vi "PositionerCapture.vi"() -> ()   [LabVIEW 2011]
doc: "CONEX - CC Virtual Front Panel:\n\nThis is a sample of an application that can be built with the LabVIEW drivers.\n\nPress HOME / ENABLE in top left of panel to put stage in Ready state for motion."
uses:
  <vilib>/userDefined/High Color/IMAQdx.ctl
  <vilib>/Platform/TimedLoop/XDataNode/timing_clust.ctl
  <vilib>/Platform/TimedLoop/XDataNode/nitl_modes.ctl
  <vilib>/Platform/TimedLoop/XDataNode/wakeup.ctl
  <vilib>/Platform/TimedLoop/XDataNode/XDataNode.xnode
  <vilib>/Platform/TimedLoop/XDataNode/XDNodeRunTimeDep.lvlib
  <vilib>/vision/driver/NI_Vision_Acquisition_Software.lvlib
panel:
  out "Current noUnits":dbl caption="mm" format="%#_6f"
  in  "lambda":dbl caption="nm" format="%#_6f"
  in  "Units":string(combo)="mm"
  in  "Go0":bool
  in  "Zero position":dbl caption="um" format="%#_6f"
  in  "Tare":bool
  out "Relative position":dbl caption="um" format="%#_6f"
  in  "Path to save the captures":path
  out "Image":T1(plugin-control)
  in  "(1) Go to:":dbl=1.0 caption="um"
  out "Title":string
  in  "Set Max":bool
  in  "Set Min":bool
  in  "Max":dbl
  in  "Min":dbl
  in  "Set velocity":bool
  out "Stop cycle":bool=TRUE
  out "Title 2":string
  in  "Cycle":bool
  in  "Go2":bool
  in  "Go1":bool
  in  "(2) Go to:":dbl=1.0 caption="um"
  in  "-":bool
  in  "+":bool
  in  "Step:":dbl caption="um" format="%#_6f"
  out "Position History":dbl(graph)=1.5
  in  "Action":bool
  out "Stop polling":bool=TRUE
  out "Controller state description":string="STATUS"
  out "Velocity MAX":dbl=0.4
  out "Controller state":string="33"
  out "Positioner error":string="0000"
  in  "Velocity:":dbl format="%#_6f"
  in  "Exit":bool=TRUE
  out "Target position":dbl
  in  "Exit":bool
  in  "Position glissière":cluster{dbl, dbl}(slide) scale=4.5..6.0
  out "Current position":dbl caption="um" format="%#_6f"
  # "mm/s"
  # "mm"
  # "Limits:"
  # "mm"
  # "(1)"
  # "(2)"
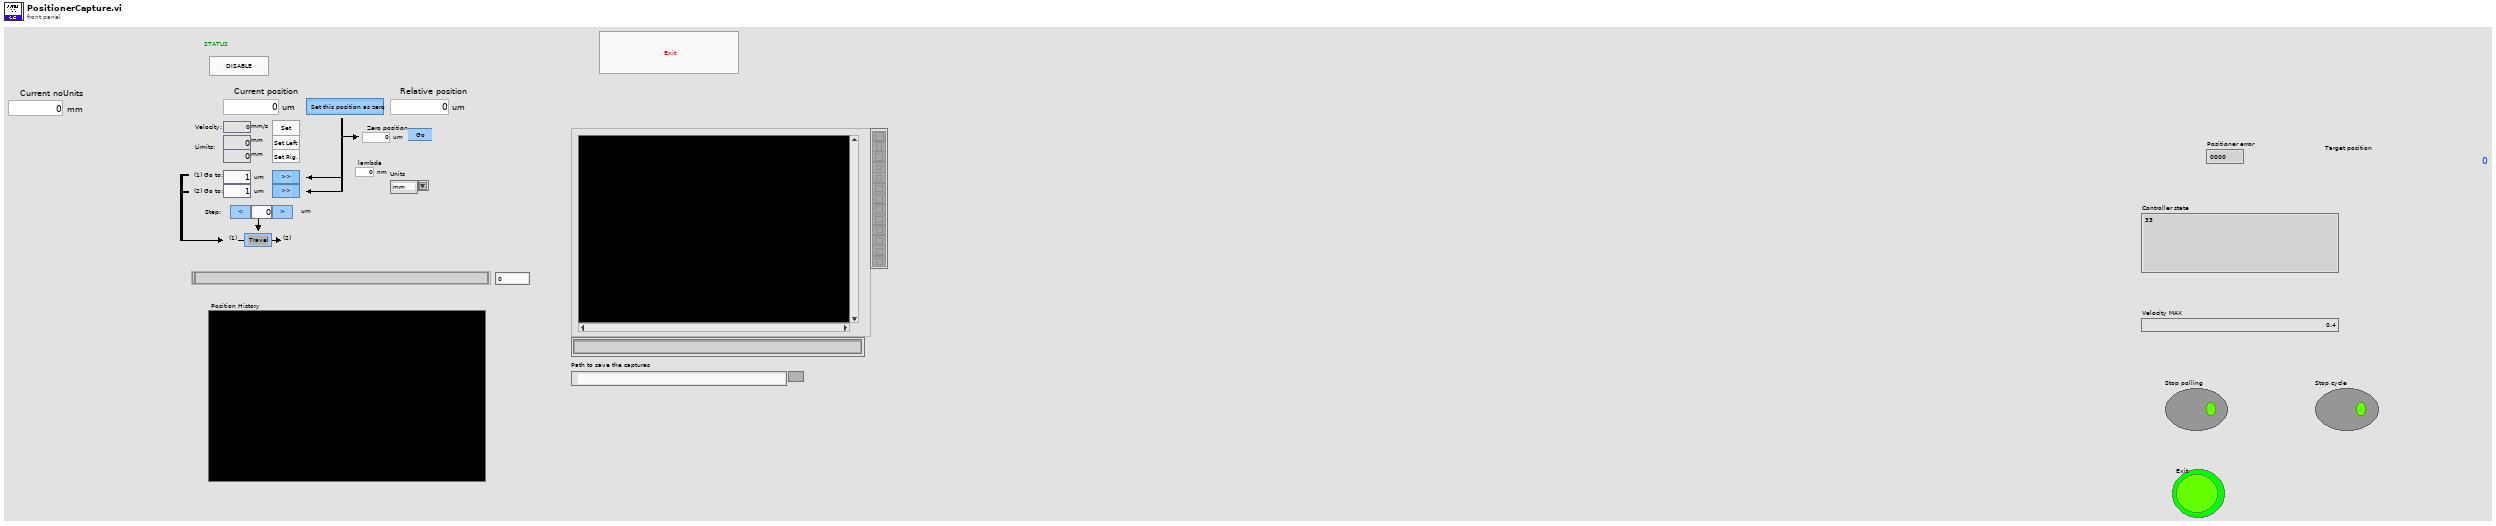
[diagram p1: front panel]
types:
  T1 = typedef "IMAQ Image.ctl" = refnum<image>
  T2 = typedef "IMAQdx.ctl" = refnum<k21>
  T3 = typedef "XDNodeRunTimeDep.lvlib/timing_clust.ctl" = cluster{"Expected End [f-1]":u64, "Actual End [f-1]":u64, "Finished Late? [f-1]":bool, "Expected End [i-1]":u64, "Actual End [i-1]":u64, "Finished Late? [i-1]":bool, "Expected Start [i]":u64, "Actual Start [i]":u64, "Expected Start [f]":u64, "Actual Start [f]":u64, "Source Name":string, "Structure Name":string, "Period":i64, "Deadline":i64, "Offset":i64, "Start":i64, "Priority":i32, "Timeout":i32, "Mode":T4, "Wakeup Reason":T5, "Error":errorcluster, "Source Type":string, "Secondary Source Type":string, "Global End Time":u64, "Global Start Time":u64, "Frame Duration":u64, "Iteration Duration":u64, "Assigned CPU":i32, "I/O Scan Engine Mode":u32}
  T4 = typedef "XDNodeRunTimeDep.lvlib/nitl_modes.ctl" = enum32{"No Change", "Process missed periods, maintain original phase", "Discard missed periods, maintain original phase", "Process missed periods, ignore original phase", "Discard missed periods, ignore original phase"}
  T5 = typedef "XDNodeRunTimeDep.lvlib/wakeup.ctl" = enum32{"Normal", "Aborted", "Asynchronous wakeup", "Timing source error", "Timed loop error", "Timeout"}
  T6 = cluster{"VISA resource name":refnum<visa-resource-name>, "Device name":string, "Controller address":i32, "error":errorcluster}
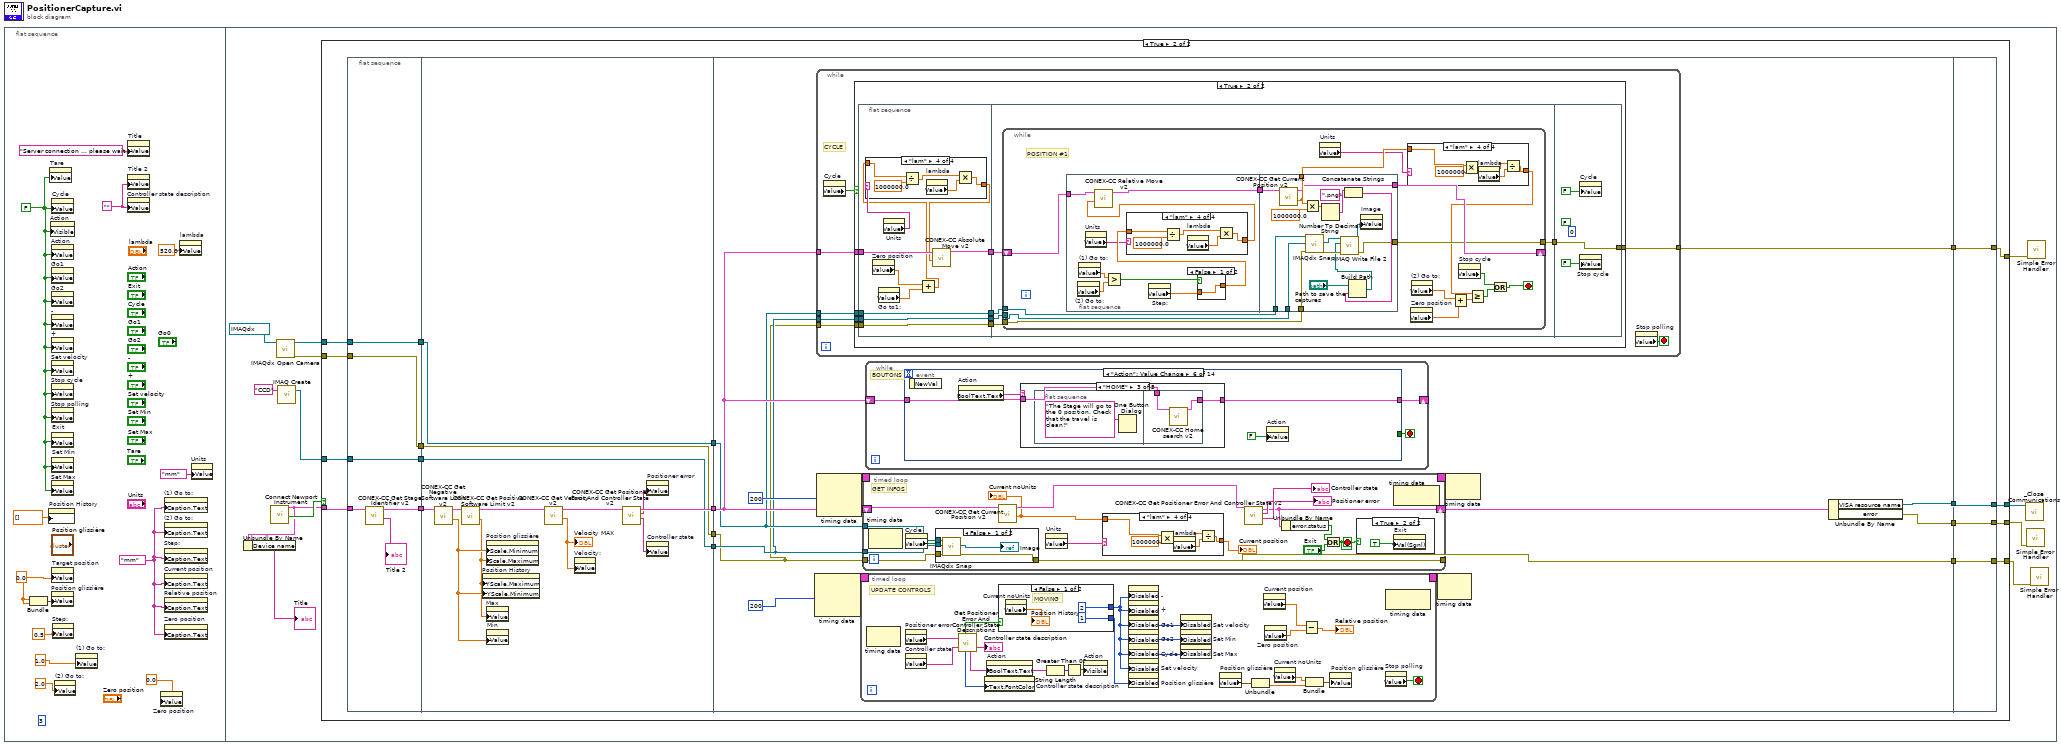
[diagram p0: block diagram]
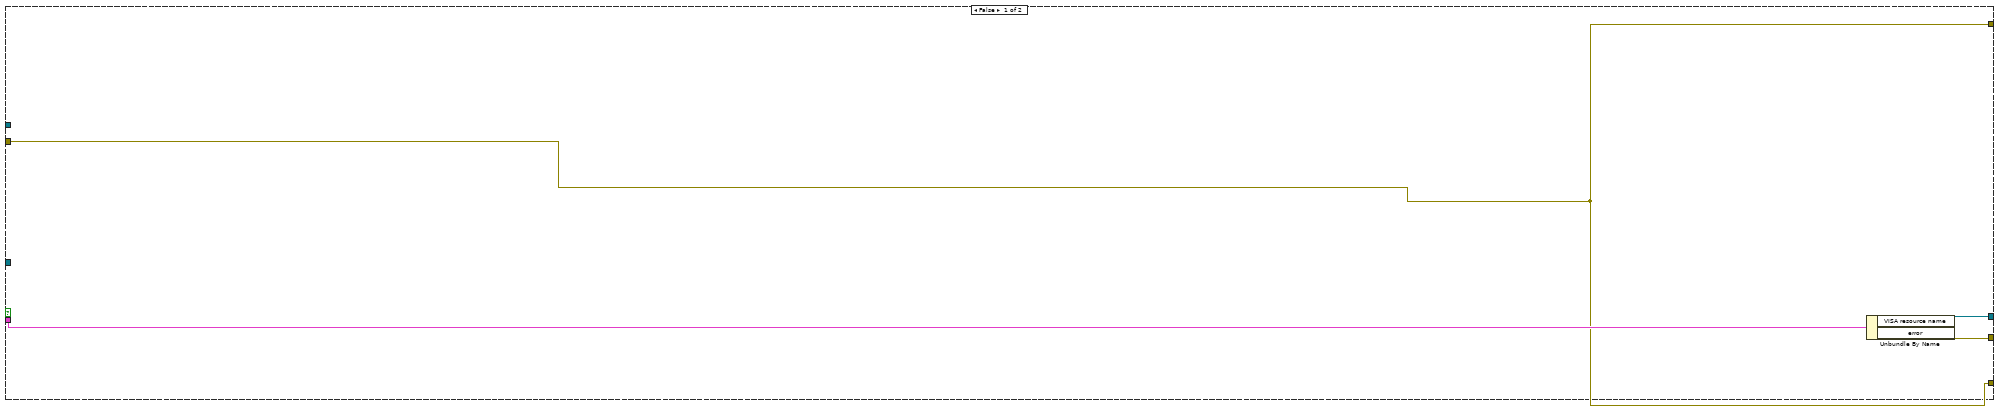
[diagram p2: hidden frame]
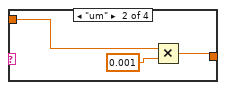
[diagram p5: hidden frame]
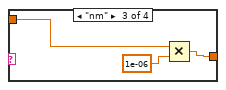
[diagram p6: hidden frame]
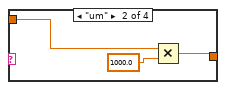
[diagram p8: hidden frame]
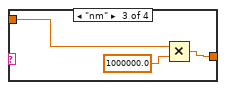
[diagram p9: hidden frame]
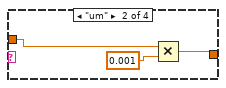
[diagram p11: hidden frame]
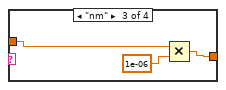
[diagram p12: hidden frame]
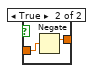
[diagram p13: hidden frame]
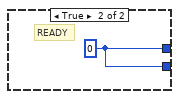
[diagram p14: hidden frame]
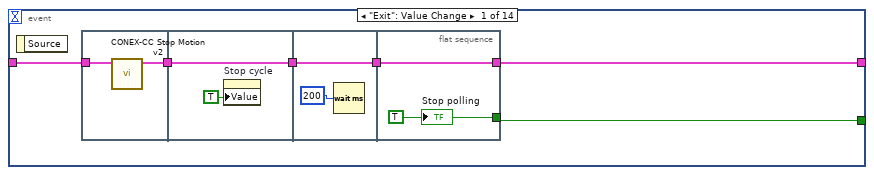
[diagram p15: hidden frame]
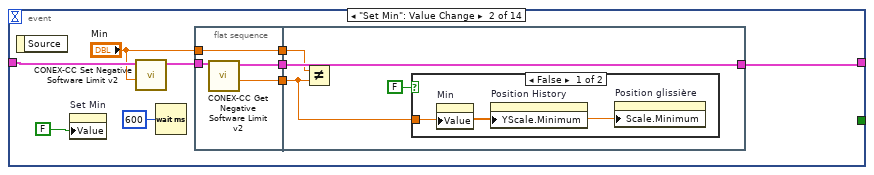
[diagram p16: hidden frame]
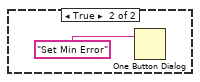
[diagram p17: hidden frame]
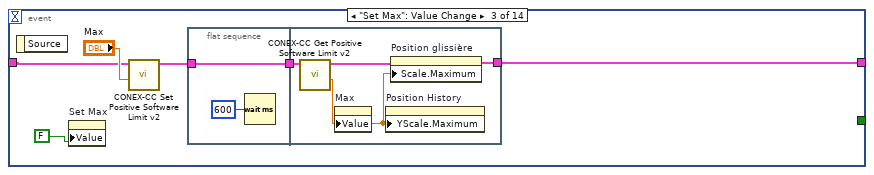
[diagram p18: hidden frame]
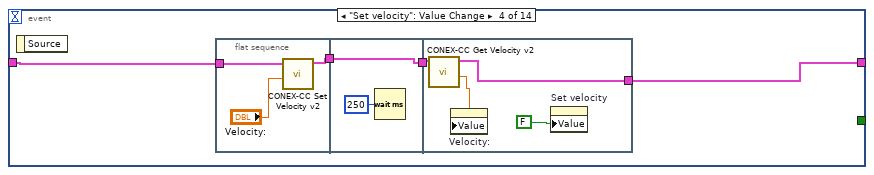
[diagram p19: hidden frame]
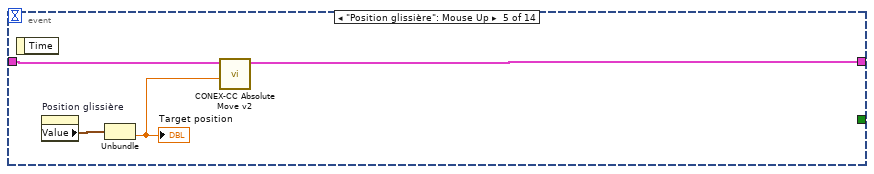
[diagram p20: hidden frame]
diagram:
  n1 = flat-sequence {
    frame #0 {
      w2 = "mm" ("Units")
      (unwired) 3 ("# Loops")
      w6 = FALSE
      w12 = 0.0
      w11 = ""
      n2 = Bundle(w12, w12) -> (w13:cluster{dbl, dbl})  [unwired: 1 out]
      n3 = property on="Position History" class="WFChart (strict)"("History Data"=dbl[] [] ("Données d'historique")) -> ()  [unwired: 2 in, 2 out]
      n4 = property on="Tare" class="Bool (strict)"("Value"=w6) -> ()  [unwired: 2 in, 2 out]
      n5 = property on="Action" class="Bool (strict)"("Visible"=w6) -> ()  [unwired: 2 in, 2 out]
      n6 = property on="Cycle" class="Bool (strict)"("Value"=w6) -> ()  [unwired: 2 in, 2 out]
      n7 = property on="Action" class="Bool (strict)"("Value"=w6) -> ()  [unwired: 2 in, 2 out]
      n8 = property on="Go1" class="Bool (strict)"("Value"=w6) -> ()  [unwired: 2 in, 2 out]
      n9 = property on="Go2" class="Bool (strict)"("Value"=w6) -> ()  [unwired: 2 in, 2 out]
      n10 = property on="-" class="Bool (strict)"("Value"=w6) -> ()  [unwired: 2 in, 2 out]
      n11 = property on="+" class="Bool (strict)"("Value"=w6) -> ()  [unwired: 2 in, 2 out]
      n12 = property on="Set velocity" class="Bool (strict)"("Value"=w6) -> ()  [unwired: 2 in, 2 out]
      n13 = property on="Stop cycle" class="Bool (strict)"("Value"=w6) -> ()  [unwired: 2 in, 2 out]
      n14 = property on="Stop polling" class="Bool (strict)"("Value"=w6) -> ()  [unwired: 2 in, 2 out]
      n15 = property on="Exit" class="Bool (strict)"("Value"=w6) -> ()  [unwired: 2 in, 2 out]
      n16 = property on="Set Min" class="Bool (strict)"("Value"=w6) -> ()  [unwired: 2 in, 2 out]
      n17 = property on="Set Max" class="Bool (strict)"("Value"=w6) -> ()  [unwired: 2 in, 2 out]
      n18 = property on="Target position" class="DigNum (strict)"("Value"=w12) -> ()  [unwired: 2 in, 2 out]
      n19 = property on="Position glissière" class="Slide (strict)"("Value"=w13) -> ()  [unwired: 2 in, 2 out]
      n20 = property on="Step:" class="DigNum (strict)"("Value"=0.5 ("Step")) -> ()  [unwired: 2 in, 2 out]
      n21 = property on="(2) Go to:" class="DigNum (strict)"("Value"=2.0 ("Abs. Move 2")) -> ()  [unwired: 2 in, 2 out]
      n22 = property on="(1) Go to:" class="DigNum (strict)"("Value"=1.0 ("Abs. Move 1")) -> ()  [unwired: 2 in, 2 out]
      n23 = property on="Title" class="Str"("Value"="Server connection ... please wait." ("Title")) -> ()  [unwired: 2 in, 2 out]
      n24 = property on="Title 2" class="Str"("Value"=w11) -> ()  [unwired: 2 in, 2 out]
      n25 = property on="Controller state description" class="Str"("Value"=w11) -> ()  [unwired: 2 in, 2 out]
      n26 = property on="Zero position" class="DigNum (strict)"("Value"=0.0 ("Zero position")) -> ()  [unwired: 2 in, 2 out]
      n27 = property on="(1) Go to:" class="DigNum (strict)"("Caption.Text"=w2) -> ()  [unwired: 2 in, 2 out]
      n28 = property on="(2) Go to:" class="DigNum (strict)"("Caption.Text"=w2) -> ()  [unwired: 2 in, 2 out]
      n29 = property on="Step:" class="DigNum (strict)"("Caption.Text"=w2) -> ()  [unwired: 2 in, 2 out]
      n30 = property on="Current position" class="DigNum (strict)"("Caption.Text"=w2) -> ()  [unwired: 2 in, 2 out]
      n31 = property on="Relative position" class="DigNum (strict)"("Caption.Text"=w2) -> ()  [unwired: 2 in, 2 out]
      n32 = property on="Zero position" class="DigNum (strict)"("Caption.Text"=w2) -> ()  [unwired: 2 in, 2 out]
      n33 = property on="lambda" class="DigNum (strict)"("Value"=520.0 ("lambda")) -> ()  [unwired: 2 in, 2 out]
      n34 = property on="Units" class="CmbBox"("Value"="mm" ("Units")) -> ()  [unwired: 2 in, 2 out]
    }
    frame #1 {
      n35 = call <userlib>:"Connect Newport Instrument.vi"() -> ("Connected"=w23:bool, "Device Connection Cluster"=w22:T6)  [unwired: 7 in, 3 out]
      n36 = Unbundle By Name(w22) -> ("Device name"=→"Title":string)
      n37 = call <vilib>:"IMAQdx Open Camera.vi"("Session In"=T2 "Paraxial") -> ("error out"=w16:errorcluster, "Session Out"=w18:T2)  [unwired: 9 in]
      n38 = call "IMAQ Create"("Image Name"="CCD") -> ("New Image"=w17:T1)  [unwired: 4 in, 1 out]
      n39 = case shown="True" w23 {
        tunnel: [w28 w49] -> w25
        tunnel: w22 -> [w29 w47]
        tunnel: [w27 w43] -> w21
        tunnel: w18 -> [_ w41]
        tunnel: w17 -> [_ w38]
        tunnel: w16 -> [w26 w35]
        tunnel: [w26 w32] -> w15
        tunnel: [w26 w30] -> w14
        frame False {
          n40 = Unbundle By Name(w29) -> ("VISA resource name"=w27:refnum<visa-resource-name>, "error"=w28:errorcluster)
        }
        frame True {
          n41 = flat-sequence {
            tunnel: w47 -> [w55]
            tunnel: [w53] -> w46
            tunnel: [w52] -> w42
            tunnel: w41 -> [w52]
            tunnel: [w51] -> w39
            tunnel: w38 -> [w51]
            tunnel: [w50] -> w36
            tunnel: w35 -> [w50]
            tunnel: [w65] -> w48
            tunnel: w46 -> [w62]
            tunnel: w42 -> [w58]
            tunnel: [w58] -> w40
            tunnel: w39 -> [w57]
            tunnel: [w57] -> w37
            tunnel: w36 -> [w56]
            tunnel: [w56] -> w34
            tunnel: w48 -> [w74]
            tunnel: [w76] -> w45
            tunnel: [w75] -> w44
            tunnel: w40 -> [w73]
            tunnel: w37 -> [w72]
            tunnel: w34 -> [w71]
            tunnel: [w70] -> w33
            tunnel: [w69] -> w31
            tunnel: [w473] -> w49
            tunnel: w45 -> [w472]
            tunnel: w44 -> [w473]
            tunnel: [w472] -> w43
            tunnel: [w471] -> w32
            tunnel: w33 -> [w471]
            tunnel: [w470] -> w30
            tunnel: w31 -> [w470]
            frame #0 {
              n42 = call <userlib>:"CONEX-CC Get Stage Identifier v2.vi"("Connection Cluster in"=w55) -> ("Identifier"=→"Title 2":string, "Connection Cluster out"=w53:T6)  [unwired: 9 in]
            }
            frame #1 {
              n43 = call <userlib>:"CONEX-CC Get Negative Software Limit v2.vi"("Connection Cluster in"=w62) -> ("Left limit"=w67:dbl, "Connection Cluster out"=w61:T6)  [unwired: 9 in]
              n44 = call <userlib>:"CONEX-CC Get Positive Software Limit v2.vi"("Connection Cluster in"=w61) -> ("Right limit"=w66:dbl, "Connection Cluster out"=w60:T6)  [unwired: 9 in]
              n45 = property on="Position History" class="WFChart (strict)"("YScale.Maximum"=w66, "YScale.Minimum"=w67) -> ()  [unwired: 2 in, 2 out]
              n46 = property on="Position glissière" class="Slide (strict)"("Scale.Minimum"=w67, "Scale.Maximum"=w66) -> ()  [unwired: 2 in, 2 out]
              n47 = property on="Max" class="DigNum (strict)"("Value"=w66) -> ()  [unwired: 2 in, 2 out]
              n48 = property on="Min" class="DigNum (strict)"("Value"=w67) -> ()  [unwired: 2 in, 2 out]
              n49 = call <userlib>:"CONEX-CC Get Velocity v2.vi"("Connection Cluster in"=w60) -> ("Velocity"=w68:dbl, "Connection Cluster out"=w59:T6)  [unwired: 8 in, 1 out]
              "Velocity MAX" <- w68
              n50 = property on="Velocity:" class="DigNum (strict)"("Value"=w68) -> ()  [unwired: 2 in, 2 out]
              n51 = call <userlib>:"CONEX-CC Get Positioner Error And Controller State v2.vi"("Connection Cluster in"=w59) -> ("Controller state"=w63:string, "Positioner error"=w64:string, "Connection Cluster out"=w65:T6)  [unwired: 8 in]
              n52 = property on="Positioner error" class="Str"("Value"=w64) -> ()  [unwired: 2 in, 2 out]
              n53 = property on="Controller state" class="Str"("Value"=w63) -> ()  [unwired: 2 in, 2 out]
            }
            frame #2 {
              n54 = node-c288(i64 200 ("Période")) -> (w81:T3)  [unwired: 1 in, 1 out]
              n55 = while {
                tunnel: w74 -> [w90]
                tunnel: w73 -> [w87]
                tunnel: w72 -> [w86]
                tunnel: w71 -> [w85]
                tunnel: [w84] -> w69
                stop <- w89 stop-if-true
                # "CYCLE"
                n56 = property on="Cycle" class="Bool (strict)"() -> ("Value"=w88:bool)  [unwired: 2 in, 2 out]
                n57 = case shown="True" w88 {
                  tunnel: w90 -> [_ w101]
                  tunnel: w87 -> [_ w98]
                  tunnel: w86 -> [_ w96]
                  tunnel: w85 -> [w91 w94]
                  tunnel: [w91 w93] -> w84
                  frame False {
                  }
                  frame True {
                    n58 = flat-sequence {
                      tunnel: w101 -> [w111]
                      tunnel: [w110] -> w100
                      tunnel: [w109] -> w99
                      tunnel: w98 -> [w109]
                      tunnel: [w108] -> w97
                      tunnel: w96 -> [w108]
                      tunnel: [w107] -> w95
                      tunnel: w94 -> [w107]
                      tunnel: w100 -> [w128]
                      tunnel: w99 -> [w127]
                      tunnel: w97 -> [w126]
                      tunnel: w95 -> [w125]
                      tunnel: [w124] -> w92
                      tunnel: [w198] -> w93
                      tunnel: w92 -> [w198]
                      frame #0 {
                        n59 = property on="Zero position" class="DigNum (strict)"() -> ("Value"=w102:dbl)  [unwired: 2 in, 2 out]
                        n60 = property on="Go to1:" class="DigNum (strict)"() -> ("Value"=w104:dbl)  [unwired: 2 in, 2 out]
                        n61 = property on="Units" class="CmbBox"() -> ("Value"=w105:string)  [unwired: 2 in, 2 out]
                        n62 = Add(x=w102, y=w104) -> (x+y=w103:dbl)
                        n63 = case shown="\"lam\"" w105 {
                          tunnel: [w112 w113 w116 w119] -> w106
                          tunnel: w103 -> [w112 w114 w117 w123]
                          frame "mm", Default {
                          }
                          frame "um" {
                            n64 = Multiply(x=w114, y=0.001) -> (x*y=w113:dbl)
                          }
                          frame "nm" {
                            n65 = Multiply(x=w117, y=1e-06) -> (x*y=w116:dbl)
                          }
                          frame "lam" {
                            n66 = Divide(x=w123, y=1000000.0) -> (x/y=w121:dbl)
                            n67 = property on="lambda" class="DigNum (strict)"() -> ("Value"=w120:dbl)  [unwired: 2 in, 2 out]
                            n68 = Multiply(x=w121, y=w120) -> (x*y=w119:dbl)
                          }
                        }
                        n69 = call <userlib>:"CONEX-CC Absolute Move v2.vi"("Target position"=w106, "Connection Cluster in"=w111) -> ("Connection Cluster out"=w110:T6)  [unwired: 5 in, 2 out]
                      }
                      frame #1 {
                        n70 = while {
                          shift-right: [w137] -> _
                          shift-left: w128 -> [w143]
                          tunnel: w127 -> [w139]
                          tunnel: w126 -> [w138]
                          tunnel: w125 -> [w140]
                          tunnel: [w136] -> w124
                          stop <- w144 stop-if-true
                          # "POSITION #1"
                          n71 = flat-sequence {
                            tunnel: w143 -> [w165]
                            tunnel: [w164] -> w135
                            tunnel: w139 -> [w197]
                            tunnel: w138 -> [w196]
                            tunnel: w140 -> [w195]
                            tunnel: w135 -> [w191]
                            tunnel: [w183] -> w134
                            tunnel: [w182] -> w137
                            tunnel: [w181] -> w136
                            frame #0 {
                              n72 = property on="(2) Go to:" class="DigNum (strict)"() -> ("Value"=w163:dbl)  [unwired: 2 in, 2 out]
                              n73 = property on="(1) Go to:" class="DigNum (strict)"() -> ("Value"=w162:dbl)  [unwired: 2 in, 2 out]
                              n74 = property on="Units" class="CmbBox"() -> ("Value"=w157:string)  [unwired: 2 in, 2 out]
                              n75 = Greater?(x=w162, y=w163) -> (0:w161:bool)
                              n76 = property on="Step:" class="DigNum (strict)"() -> ("Value"=w160:dbl)  [unwired: 2 in, 2 out]
                              n77 = case shown="False" w161 {
                                tunnel: [w178 w179] -> w159
                                tunnel: w160 -> [w178 w180]
                                frame False {
                                }
                                frame True {
                                n78 = Negate(x=w180) -> (-x=w179:dbl)
                                }
                              }
                              n79 = case shown="\"lam\"" w157 {
                                tunnel: [w166 w168 w171 w174] -> w158
                                tunnel: w159 -> [w166 w167 w170 w173]
                                frame "mm", Default {
                                }
                                frame "um" {
                                n80 = Multiply(x=w167, y=0.001) -> (x*y=w168:dbl)
                                }
                                frame "nm" {
                                n81 = Multiply(x=w170, y=1e-06) -> (x*y=w171:dbl)
                                }
                                frame "lam" {
                                n82 = Divide(x=w173, y=1000000.0) -> (x/y=w176:dbl)
                                n83 = property on="lambda" class="DigNum (strict)"() -> ("Value"=w175:dbl)  [unwired: 2 in, 2 out]
                                n84 = Multiply(x=w176, y=w175) -> (x*y=w174:dbl)
                                }
                              }
                              n85 = call <userlib>:"CONEX-CC Relative Move v2.vi"("Relative displacement"=w158, "Connection Cluster in"=w165) -> ("Connection Cluster out"=w164:T6)  [unwired: 9 in]
                            }
                            frame #1 {
                              n86 = call <userlib>:"CONEX-CC Get Current Position v2.vi"("Connection Cluster in"=w191) -> ("Current position"=w183:dbl, "Connection Cluster out"=w182:T6)  [unwired: 8 in, 1 out]
                              n87 = Multiply(x=w183, y=1000000.0) -> (x*y=w187:dbl)
                              n88 = call <vilib>:"IMAQdx Snap.vi"("error in"=w195, "Image In"=w196, "Session In"=w197) -> ("error out"=w193:errorcluster, "Image Out"=w194:T1)  [unwired: 6 in, 1 out]
                              n89 = Number To Decimal String(number=w187) -> (decimal integer string=w186:string)  [unwired: 1 in]
                              n90 = Concatenate Strings(w186, ".png" ("string")) -> (w184:string)
                              n91 = Build Path(base path="Path to save the captures", name or relative path=w184) -> (appended path=w188:path)
                              n92 = call-poly "IMAQ Write File 2"("error in (no error)"=w193, "File Path"=w188, "Image"=w194) -> ("error out"=w181:errorcluster, "Image Out (duplicate)"=w192:T1)  [unwired: 7 in]
                              n93 = property on="Image" class="ImageControl"("Value"=w192) -> ()  [unwired: 2 in, 2 out]
                            }
                          }
                          n94 = property on="Units" class="CmbBox"() -> ("Value"=w132:string)  [unwired: 2 in, 2 out]
                          n95 = case shown="\"lam\"" w132 {
                            tunnel: [w145 w146 w149 w152] -> w133
                            tunnel: w134 -> [w145 w147 w150 w153]
                            frame "mm", Default {
                            }
                            frame "um" {
                              n96 = Multiply(x=w147, y=1000.0) -> (x*y=w146:dbl)
                            }
                            frame "nm" {
                              n97 = Multiply(x=w150, y=1000000.0) -> (x*y=w149:dbl)
                            }
                            frame "lam" {
                              n98 = Multiply(x=w153, y=1000000.0) -> (x*y=w156:dbl)
                              n99 = property on="lambda" class="DigNum (strict)"() -> ("Value"=w154:dbl)  [unwired: 2 in, 2 out]
                              n100 = Divide(x=w156, y=w154) -> (x/y=w152:dbl)
                            }
                          }
                          n101 = property on="Zero position" class="DigNum (strict)"() -> ("Value"=w129:dbl)  [unwired: 2 in, 2 out]
                          n102 = property on="(2) Go to:" class="DigNum (strict)"() -> ("Value"=w130:dbl)  [unwired: 2 in, 2 out]
                          n103 = Add(x=w130, y=w129) -> (x+y=w131:dbl)
                          n104 = property on="Stop cycle" class="Bool (strict)"() -> ("Value"=w141:bool)  [unwired: 2 in, 2 out]
                          n105 = Greater Or Equal?(x=w133, y=w131) -> (x >= y?=w142:bool)
                          n106 = Or(x=w141, y=w142) -> (x .or. y?=w144:bool)
                        }
                      }
                      frame #2 {
                        (unwired) 0 ("counter")
                        (unwired) FALSE ("Visible")
                        n107 = property on="Cycle" class="Bool (strict)"("Value"=FALSE ("Cycle")) -> ()  [unwired: 2 in, 2 out]
                        n108 = property on="Stop cycle" class="Bool (strict)"("Value"=FALSE ("Cycle")) -> ()  [unwired: 2 in, 2 out]
                      }
                    }
                  }
                }
                n109 = property on="Stop polling" class="Bool (strict)"() -> ("Value"=w89:bool)  [unwired: 2 in, 2 out]
              }
              n110 = node-c288(i64 200 ("Période")) -> (w83:T3)  [unwired: 1 in, 1 out]
              n111 = timed-loop {
                timing: w81 -> [_]
                timing-out: [_] -> w80
                stop <- w209 stop-if-true
                # "UPDATE CONTROLS"
                n112 = node-c288() -> ()  [unwired: 2 out]
                n113 = property on="Positioner error" class="Str"() -> ("Value"=w218:string)  [unwired: 2 in, 2 out]
                n114 = property on="Controller state" class="Str"() -> ("Value"=w217:string)  [unwired: 2 in, 2 out]
                n115 = call <userlib>:"Get Positioner Error And Controller State Descriptions.vi"("Controller state"=w217, "Positioner error"=w218) -> ("Color"=w215:u32, "Action name"=w214:string, "Controller state description"=→"Controller state description":string, "IsReady?"=w211:bool)  [unwired: 2 out]
                n116 = property on="Controller state description" class="Str"("Text.FontColor"=w215) -> ()  [unwired: 2 in, 2 out]
                n117 = property on="Action" class="Bool (strict)"("BoolText.Text"=w214) -> ()  [unwired: 2 in, 2 out]
                n118 = case shown="False" w211 {
                  tunnel: [u8 2 w222] -> w208
                  tunnel: [u8 1 w222] -> w210
                  frame False {
                    # "MOVING"
                    n119 = property on="Current noUnits" class="DigNum (strict)"() -> ("Value"=→"Position History":dbl)  [unwired: 2 in, 2 out]
                  }
                  frame True {
                    w222 = u8 0
                    # "READY"
                  }
                }
                n120 = String Length(string=w214) -> (length=w213:i32)
                n121 = Greater Than 0?(x=w213) -> (x > 0?=w212:bool)
                n122 = property on="Action" class="Bool (strict)"("Visible"=w212) -> ()  [unwired: 2 in, 2 out]
                n123 = property on="-" class="Bool (strict)"("Disabled"=w208) -> ()  [unwired: 2 in, 2 out]
                n124 = property on="+" class="Bool (strict)"("Disabled"=w208) -> ()  [unwired: 2 in, 2 out]
                n125 = property on="Go1" class="Bool (strict)"("Disabled"=w208) -> ()  [unwired: 2 in, 2 out]
                n126 = property on="Go2" class="Bool (strict)"("Disabled"=w208) -> ()  [unwired: 2 in, 2 out]
                n127 = property on="Cycle" class="Bool (strict)"("Disabled"=w208) -> ()  [unwired: 2 in, 2 out]
                n128 = property on="Set velocity" class="Bool (strict)"("Disabled"=w208) -> ()  [unwired: 2 in, 2 out]
                n129 = property on="Position glissière" class="Slide (strict)"("Disabled"=w210) -> ()  [unwired: 2 in, 2 out]
                n130 = property on="Set velocity" class="Bool (strict)"("Disabled"=w208) -> ()  [unwired: 2 in, 2 out]
                n131 = property on="Set Min" class="Bool (strict)"("Disabled"=w208) -> ()  [unwired: 2 in, 2 out]
                n132 = property on="Set Max" class="Bool (strict)"("Disabled"=w208) -> ()  [unwired: 2 in, 2 out]
                n133 = property on="Position glissière" class="Slide (strict)"() -> ("Value"=w206:cluster{dbl, dbl})  [unwired: 2 in, 2 out]
                n134 = Unbundle(w206) -> (w205:dbl)  [unwired: 1 out]
                n135 = property on="Current position" class="DigNum (strict)"() -> ("Value"=w201:dbl)  [unwired: 2 in, 2 out]
                n136 = property on="Zero position" class="DigNum (strict)"() -> ("Value"=w202:dbl)  [unwired: 2 in, 2 out]
                n137 = property on="Current noUnits" class="DigNum (strict)"() -> ("Value"=w203:dbl)  [unwired: 2 in, 2 out]
                n138 = Subtract(x=w201, y=w202) -> (x-y=→"Relative position":dbl)
                n139 = Bundle("Value"=w203, w205) -> (w207:cluster{"Value":dbl, dbl})  [unwired: 1 out]
                n140 = property on="Position glissière" class="Slide (strict)"("Value"=w207) -> ()  [unwired: 2 in, 2 out]
                n141 = node-c288() -> ()  [unwired: 2 out]
                n142 = property on="Stop polling" class="Bool (strict)"() -> ("Value"=w209:bool)  [unwired: 2 in, 2 out]
              }
              n143 = timed-loop {
                timing: w83 -> [_]
                timing-out: [_] -> w82
                shift-right: [w434] -> w77
                shift-left: w74 -> [w444]
                tunnel: w73 -> [w443]
                tunnel: w72 -> [w442]
                tunnel: w71 -> [w441]
                tunnel: [w440] -> w70
                stop <- w437 stop-if-true
                # "GET INFOS"
                n144 = node-c288() -> ()  [unwired: 2 out]
                n145 = property on="Cycle" class="Bool (strict)"() -> ("Value"=w439:bool)  [unwired: 2 in, 2 out]
                n146 = case shown="False" w439 {
                  tunnel: w443 -> [w461 _]
                  tunnel: w442 -> [w460 _]
                  tunnel: w441 -> [w459 w462]
                  tunnel: [w457 w462] -> w440
                  frame False {
                    n147 = call <vilib>:"IMAQdx Snap.vi"("error in"=w459, "Image In"=w460, "Session In"=w461) -> ("error out"=w457:errorcluster, "Image Out"=→"Image":T1)  [unwired: 6 in, 1 out]
                  }
                  frame True {
                  }
                }
                n148 = call <userlib>:"CONEX-CC Get Current Position v2.vi"("Connection Cluster in"=w444) -> ("Current position"=w430:dbl, "Connection Cluster out"=w431:T6)  [unwired: 8 in, 1 out]
                "Current noUnits" <- w430
                n149 = property on="Units" class="CmbBox"() -> ("Value"=w429:string)  [unwired: 2 in, 2 out]
                n150 = case shown="\"lam\"" w429 {
                  tunnel: [w445 w446 w449 w452] -> w433
                  tunnel: w430 -> [w445 w447 w450 w453]
                  frame "mm", Default {
                  }
                  frame "um" {
                    n151 = Multiply(x=w447, y=1000.0) -> (x*y=w446:dbl)
                  }
                  frame "nm" {
                    n152 = Multiply(x=w450, y=1000000.0) -> (x*y=w449:dbl)
                  }
                  frame "lam" {
                    n153 = Multiply(x=w453, y=1000000.0) -> (x*y=w456:dbl)
                    n154 = property on="lambda" class="DigNum (strict)"() -> ("Value"=w454:dbl)  [unwired: 2 in, 2 out]
                    n155 = Divide(x=w456, y=w454) -> (x/y=w452:dbl)
                  }
                }
                "Current position" <- w433
                n156 = call <userlib>:"CONEX-CC Get Positioner Error And Controller State v2.vi"("Connection Cluster in"=w431) -> ("Controller state"=→"Controller state":string, "Positioner error"=→"Positioner error":string, "Connection Cluster out"=w434:T6)  [unwired: 8 in]
                n157 = Unbundle By Name(w434) -> ("error.status"=w432:bool)
                n158 = Or(x=w432, y="Exit") -> (x .or. y?=w437:bool)
                n159 = case shown="True" w437 {
                  frame False {
                  }
                  frame True {
                    n160 = property on="Exit" class="Bool (strict)"("Val(Sgnl)"=TRUE) -> ()  [unwired: 2 in, 2 out]
                  }
                }
                n161 = node-c288() -> ()  [unwired: 2 out]
              }
              n162 = while {
                shift-right: [w231] -> _
                shift-left: w74 -> [w230]
                stop <- w229 stop-if-true
                # "BOUTONS"
                n163 = event shown="[5] \"Action\": Value Change" {
                  selector: _ -> [_ _ _ _ _ _ _ _ _ _ _ _ _ _]
                  dyn-events: _ -> [_ _ _ _ _ _ _ _ _ _ _ _ _ _]
                  timeout: _ -> [_ _ _ _ _ _ _ _ _ _ _ _ _ _]
                  tunnel: [w235 _ _ _ _ _ _ _ _ _ _ _ _ _] -> w229
                  tunnel: w230 -> [w232 w252 w266 w279 w291 w295 w314 w335 w356 w376 w393 w409 w411 w420]
                  tunnel: [w237 w251 w265 w276 w290 w294 w313 w336 w355 w375 w394 w409 w411 w420] -> w231
                  event "Exit": Value Change {
                    n164 = event-data() -> ()  [unwired: 2 out]
                    n165 = flat-sequence {
                      tunnel: [w239] -> w236
                      tunnel: w232 -> [w238]
                      tunnel: w236 -> [w241]
                      tunnel: [w241] -> w234
                      tunnel: w234 -> [w243]
                      tunnel: [w243] -> w233
                      tunnel: [w245] -> w237
                      tunnel: w233 -> [w245]
                      tunnel: [w244] -> w235
                      frame #0 {
                        n166 = call <userlib>:"CONEX-CC Stop Motion v2.vi"("Connection Cluster in"=w238) -> ("Connection Cluster out"=w239:T6)  [unwired: 10 in]
                      }
                      frame #1 {
                        n167 = property on="Stop cycle" class="Bool (strict)"("Value"=TRUE) -> ()  [unwired: 2 in, 2 out]
                      }
                      frame #2 {
                        n168 = Wait (ms)(milliseconds to wait=u32 200 ("attente (ms)")) -> ()  [unwired: 1 out]
                      }
                      frame #3 {
                        w244 = TRUE
                        "Stop polling" <- w244
                      }
                    }
                  }
                  event "Set Min": Value Change {
                    n169 = event-data() -> ()  [unwired: 2 out]
                    n170 = property on="Set Min" class="Bool (strict)"("Value"=FALSE ("Set Min")) -> ()  [unwired: 2 in, 2 out]
                    n171 = call <userlib>:"CONEX-CC Set Negative Software Limit v2.vi"("Negative limit (left)"="Min", "Connection Cluster in"=w252) -> ("Connection Cluster out"=w254:T6)  [unwired: 9 in]
                    n172 = Wait (ms)(milliseconds to wait=u32 600 ("attente (ms)")) -> ()  [unwired: 1 out]
                    n173 = flat-sequence {
                      tunnel: w254 -> [w258]
                      tunnel: [w257] -> w249
                      tunnel: [w256] -> w248
                      tunnel: "Min" -> [w256]
                      tunnel: [w255] -> w246
                      tunnel: [w262] -> w251
                      tunnel: w249 -> [w262]
                      tunnel: w248 -> [w261]
                      tunnel: w246 -> [w259]
                      frame #0 {
                        n174 = call <userlib>:"CONEX-CC Get Negative Software Limit v2.vi"("Connection Cluster in"=w258) -> ("Left limit"=w255:dbl, "Connection Cluster out"=w257:T6)  [unwired: 9 in]
                      }
                      frame #1 {
                        n175 = Not Equal?(x=w261, y=w259) -> ()  [unwired: 1 out]
                        n176 = case shown="False" FALSE {
                          tunnel: w259 -> [w263 _]
                          frame False {
                            n177 = property on="Min" class="DigNum (strict)"("Value"=w263) -> ()  [unwired: 2 in, 2 out]
                            n178 = property on="Position History" class="WFChart (strict)"("YScale.Minimum"=w263) -> ()  [unwired: 2 in, 2 out]
                            n179 = property on="Position glissière" class="Slide (strict)"("Scale.Minimum"=w263) -> ()  [unwired: 2 in, 2 out]
                          }
                          frame True {
                            n180 = One Button Dialog(message="Set Min Error") -> ()  [unwired: 1 in, 1 out]
                          }
                        }
                      }
                    }
                  }
                  event "Set Max": Value Change {
                    n181 = event-data() -> ()  [unwired: 2 out]
                    n182 = property on="Set Max" class="Bool (strict)"("Value"=FALSE ("Set Max")) -> ()  [unwired: 2 in, 2 out]
                    n183 = call <userlib>:"CONEX-CC Set Positive Software Limit v2.vi"("Positive limit (right)"="Max", "Connection Cluster in"=w266) -> ("Connection Cluster out"=w270:T6)  [unwired: 9 in]
                    n184 = flat-sequence {
                      tunnel: w270 -> [w272]
                      tunnel: [w272] -> w267
                      tunnel: [w275] -> w265
                      tunnel: w267 -> [w273]
                      frame #0 {
                        n185 = Wait (ms)(milliseconds to wait=u32 600 ("attente (ms)")) -> ()  [unwired: 1 out]
                      }
                      frame #1 {
                        n186 = call <userlib>:"CONEX-CC Get Positive Software Limit v2.vi"("Connection Cluster in"=w273) -> ("Right limit"=w274:dbl, "Connection Cluster out"=w275:T6)  [unwired: 9 in]
                        n187 = property on="Max" class="DigNum (strict)"("Value"=w274) -> ()  [unwired: 2 in, 2 out]
                        n188 = property on="Position History" class="WFChart (strict)"("YScale.Maximum"=w274) -> ()  [unwired: 2 in, 2 out]
                        n189 = property on="Position glissière" class="Slide (strict)"("Scale.Maximum"=w274) -> ()  [unwired: 2 in, 2 out]
                      }
                    }
                  }
                  event "Set velocity": Value Change {
                    n190 = event-data() -> ()  [unwired: 2 out]
                    n191 = flat-sequence {
                      tunnel: w279 -> [w281]
                      tunnel: [w280] -> w277
                      tunnel: [w284] -> w278
                      tunnel: w277 -> [w284]
                      tunnel: w278 -> [w288]
                      tunnel: [w287] -> w276
                      frame #0 {
                        n192 = call <userlib>:"CONEX-CC Set Velocity v2.vi"("Velocity"="Velocity:", "Connection Cluster in"=w281) -> ("Connection Cluster out"=w280:T6)  [unwired: 9 in]
                      }
                      frame #1 {
                        n193 = Wait (ms)(milliseconds to wait=u32 250 ("attente (ms)")) -> ()  [unwired: 1 out]
                      }
                      frame #2 {
                        n194 = call <userlib>:"CONEX-CC Get Velocity v2.vi"("Connection Cluster in"=w288) -> ("Velocity"=w286:dbl, "Connection Cluster out"=w287:T6)  [unwired: 8 in, 1 out]
                        n195 = property on="Velocity:" class="DigNum (strict)"("Value"=w286) -> ()  [unwired: 2 in, 2 out]
                        n196 = property on="Set velocity" class="Bool (strict)"("Value"=FALSE ("Set velocity")) -> ()  [unwired: 2 in, 2 out]
                      }
                    }
                  }
                  event "Position glissière": Mouse Up {
                    n197 = event-data() -> ()  [unwired: 2 out]
                    n198 = property on="Position glissière" class="Slide (strict)"() -> ("Value"=w292:cluster{dbl, dbl})  [unwired: 2 in, 2 out]
                    n199 = Unbundle(w292) -> (w289:dbl)  [unwired: 1 out]
                    "Target position" <- w289
                    n200 = call <userlib>:"CONEX-CC Absolute Move v2.vi"("Target position"=w289, "Connection Cluster in"=w291) -> ("Connection Cluster out"=w290:T6)  [unwired: 5 in, 2 out]
                  }
                  event "Action": Value Change {
                    n201 = event-data() -> ()  [unwired: 2 out]
                    n202 = property on="Action" class="Bool (strict)"() -> ("BoolText.Text"=w296:string)  [unwired: 2 in, 2 out]
                    n203 = case shown="\"HOME\"" w296 {
                      tunnel: w295 -> [w298 w300 w302 w308 w310]
                      tunnel: [w297 w300 w301 w307 w312] -> w294
                      frame "ENABLE" {
                        n204 = call <userlib>:"CONEX-CC Enter-Leave DISABLE State v2.vi"("Ready? (false=DISABLE true=READY)"=TRUE ("Flag (false=DISABLE true=READY)"), "Connection Cluster in"=w298) -> ("Connection Cluster out"=w297:T6)  [unwired: 7 in]
                      }
                      frame Default {
                      }
                      frame "HOME" {
                        n205 = flat-sequence {
                          tunnel: w302 -> [w305]
                          tunnel: [w304] -> w301
                          frame #0 {
                            n206 = One Button Dialog(message="The Stage will go to the 0 position. Check that the travel is clean!") -> ()  [unwired: 1 in, 1 out]
                          }
                          frame #1 {
                            n207 = call <userlib>:"CONEX-CC Home search v2.vi"("Connection Cluster in"=w305) -> ("Connection Cluster out"=w304:T6)  [unwired: 5 in, 3 out]
                          }
                        }
                      }
                      frame "DISABLE" {
                        n208 = call <userlib>:"CONEX-CC Enter-Leave DISABLE State v2.vi"("Ready? (false=DISABLE true=READY)"=FALSE ("Flag (false=DISABLE true=READY)"), "Connection Cluster in"=w308) -> ("Connection Cluster out"=w307:T6)  [unwired: 7 in]
                      }
                      frame "STOP" {
                        n209 = call <userlib>:"CONEX-CC Stop Motion v2.vi"("Connection Cluster in"=w310) -> ("Connection Cluster out"=w312:T6)  [unwired: 10 in]
                        n210 = property on="Stop cycle" class="Bool (strict)"("Value"=TRUE) -> ()  [unwired: 2 in, 2 out]
                        "Stop cycle" <- TRUE ("Stop cycle")
                      }
                    }
                    n211 = property on="Action" class="Bool (strict)"("Value"=FALSE) -> ()  [unwired: 2 in, 2 out]
                  }
                  event "-": Value Change {
                    n212 = event-data() -> ()  [unwired: 2 out]
                    n213 = property on="-" class="Bool (strict)"("Value"=FALSE ("-")) -> ()  [unwired: 2 in, 2 out]
                    n214 = Negate(x="Step:") -> (-x=w317:dbl)
                    n215 = property on="Units" class="CmbBox"() -> ("Value"=w315:string)  [unwired: 2 in, 2 out]
                    n216 = case shown="\"lam\"" w315 {
                      tunnel: [w320 w321 w324 w327] -> w316
                      tunnel: w317 -> [w320 w322 w325 w331]
                      frame "mm", Default {
                      }
                      frame "um" {
                        n217 = Multiply(x=w322, y=0.001) -> (x*y=w321:dbl)
                      }
                      frame "nm" {
                        n218 = Multiply(x=w325, y=1e-06) -> (x*y=w324:dbl)
                      }
                      frame "lam" {
                        n219 = Divide(x=w331, y=1000000.0) -> (x/y=w329:dbl)
                        n220 = property on="lambda" class="DigNum (strict)"() -> ("Value"=w328:dbl)  [unwired: 2 in, 2 out]
                        n221 = Multiply(x=w329, y=w328) -> (x*y=w327:dbl)
                      }
                    }
                    n222 = call <userlib>:"CONEX-CC Relative Move v2.vi"("Relative displacement"=w316, "Connection Cluster in"=w314) -> ("Connection Cluster out"=w313:T6)  [unwired: 9 in]
                  }
                  event "+": Value Change {
                    n223 = event-data() -> ()  [unwired: 2 out]
                    n224 = property on="+" class="Bool (strict)"("Value"=FALSE ("+")) -> ()  [unwired: 2 in, 2 out]
                    n225 = property on="Step:" class="DigNum (strict)"() -> ("Value"=w334:dbl)  [unwired: 2 in, 2 out]
                    n226 = property on="Units" class="CmbBox"() -> ("Value"=w333:string)  [unwired: 2 in, 2 out]
                    n227 = case shown="\"lam\"" w333 {
                      tunnel: [w338 w339 w342 w345] -> w332
                      tunnel: w334 -> [w338 w340 w343 w349]
                      frame "mm", Default {
                      }
                      frame "um" {
                        n228 = Multiply(x=w340, y=0.001) -> (x*y=w339:dbl)
                      }
                      frame "nm" {
                        n229 = Multiply(x=w343, y=1e-06) -> (x*y=w342:dbl)
                      }
                      frame "lam" {
                        n230 = Divide(x=w349, y=1000000.0) -> (x/y=w347:dbl)
                        n231 = property on="lambda" class="DigNum (strict)"() -> ("Value"=w346:dbl)  [unwired: 2 in, 2 out]
                        n232 = Multiply(x=w347, y=w346) -> (x*y=w345:dbl)
                      }
                    }
                    n233 = call <userlib>:"CONEX-CC Relative Move v2.vi"("Relative displacement"=w332, "Connection Cluster in"=w335) -> ("Connection Cluster out"=w336:T6)  [unwired: 9 in]
                  }
                  event "Go1": Value Change {
                    n234 = event-data() -> ()  [unwired: 2 out]
                    n235 = property on="Go1" class="Bool (strict)"("Value"=FALSE ("Go1")) -> ()  [unwired: 2 in, 2 out]
                    n236 = property on="Zero position" class="DigNum (strict)"() -> ("Value"=w353:dbl)  [unwired: 2 in, 2 out]
                    n237 = property on="Units" class="CmbBox"() -> ("Value"=w354:string)  [unwired: 2 in, 2 out]
                    n238 = Add(x="(1) Go to:", y=w353) -> (x+y=w351:dbl)
                    n239 = case shown="\"lam\"" w354 {
                      tunnel: [w358 w359 w362 w365] -> w350
                      tunnel: w351 -> [w358 w360 w363 w369]
                      frame "mm", Default {
                      }
                      frame "um" {
                        n240 = Multiply(x=w360, y=0.001) -> (x*y=w359:dbl)
                      }
                      frame "nm" {
                        n241 = Multiply(x=w363, y=1e-06) -> (x*y=w362:dbl)
                      }
                      frame "lam" {
                        n242 = Divide(x=w369, y=1000000.0) -> (x/y=w367:dbl)
                        n243 = property on="lambda" class="DigNum (strict)"() -> ("Value"=w366:dbl)  [unwired: 2 in, 2 out]
                        n244 = Multiply(x=w367, y=w366) -> (x*y=w365:dbl)
                      }
                    }
                    n245 = call <userlib>:"CONEX-CC Absolute Move v2.vi"("Target position"=w350, "Connection Cluster in"=w356) -> ("Connection Cluster out"=w355:T6)  [unwired: 5 in, 2 out]
                  }
                  event "Go2": Value Change {
                    n246 = event-data() -> ()  [unwired: 2 out]
                    n247 = property on="Go2" class="Bool (strict)"("Value"=FALSE ("Go2")) -> ()  [unwired: 2 in, 2 out]
                    n248 = property on="Zero position" class="DigNum (strict)"() -> ("Value"=w373:dbl)  [unwired: 2 in, 2 out]
                    n249 = property on="Units" class="CmbBox"() -> ("Value"=w374:string)  [unwired: 2 in, 2 out]
                    n250 = Add(x="(2) Go to:", y=w373) -> (x+y=w371:dbl)
                    n251 = case shown="\"lam\"" w374 {
                      tunnel: [w378 w380 w383 w386] -> w370
                      tunnel: w371 -> [w378 w379 w382 w385]
                      frame "mm", Default {
                      }
                      frame "um" {
                        n252 = Multiply(x=w379, y=0.001) -> (x*y=w380:dbl)
                      }
                      frame "nm" {
                        n253 = Multiply(x=w382, y=1e-06) -> (x*y=w383:dbl)
                      }
                      frame "lam" {
                        n254 = Divide(x=w385, y=1000000.0) -> (x/y=w388:dbl)
                        n255 = property on="lambda" class="DigNum (strict)"() -> ("Value"=w387:dbl)  [unwired: 2 in, 2 out]
                        n256 = Multiply(x=w388, y=w387) -> (x*y=w386:dbl)
                      }
                    }
                    n257 = call <userlib>:"CONEX-CC Absolute Move v2.vi"("Target position"=w370, "Connection Cluster in"=w376) -> ("Connection Cluster out"=w375:T6)  [unwired: 5 in, 2 out]
                  }
                  event "Go0": Value Change {
                    n258 = event-data() -> ()  [unwired: 2 out]
                    n259 = property on="Zero position" class="DigNum (strict)"() -> ("Value"=w390:dbl)  [unwired: 2 in, 2 out]
                    n260 = property on="Go0" class="Bool (strict)"("Value"=FALSE ("Go2")) -> ()  [unwired: 2 in, 2 out]
                    n261 = property on="Units" class="CmbBox"() -> ("Value"=w391:string)  [unwired: 2 in, 2 out]
                    n262 = case shown="\"lam\"" w391 {
                      tunnel: [w396 w398 w401 w404] -> w392
                      tunnel: w390 -> [w396 w397 w400 w403]
                      frame "mm", Default {
                      }
                      frame "um" {
                        n263 = Multiply(x=w397, y=0.001) -> (x*y=w398:dbl)
                      }
                      frame "nm" {
                        n264 = Multiply(x=w400, y=1e-06) -> (x*y=w401:dbl)
                      }
                      frame "lam" {
                        n265 = Divide(x=w403, y=1000000.0) -> (x/y=w406:dbl)
                        n266 = property on="lambda" class="DigNum (strict)"() -> ("Value"=w405:dbl)  [unwired: 2 in, 2 out]
                        n267 = Multiply(x=w406, y=w405) -> (x*y=w404:dbl)
                      }
                    }
                    n268 = call <userlib>:"CONEX-CC Absolute Move v2.vi"("Target position"=w392, "Connection Cluster in"=w393) -> ("Connection Cluster out"=w394:T6)  [unwired: 5 in, 2 out]
                  }
                  event "Tare": Value Change {
                    n269 = event-data() -> ()  [unwired: 2 out]
                    n270 = property on="Tare" class="Bool (strict)"("Value"=FALSE ("Tare")) -> ()  [unwired: 2 in, 2 out]
                    n271 = property on="Current position" class="DigNum (strict)"() -> ("Value"=w408:dbl)  [unwired: 2 in, 2 out]
                    n272 = property on="Zero position" class="DigNum (strict)"("Value"=w408) -> ()  [unwired: 2 in, 2 out]
                  }
                  event "Cycle": Value Change {
                    (unwired) 0 ("Numérique")
                    n273 = event-data() -> ()  [unwired: 2 out]
                    n274 = property on="Cycle" class="Bool (strict)"("Value"=TRUE ("Cycle")) -> ()  [unwired: 2 in, 2 out]
                  }
                  event "Units": Value Change {
                    n275 = event-data() -> ("NewVal"=w419:string, "OldVal"=w418:string)  [unwired: 1 out]
                    n276 = property on="(1) Go to:" class="DigNum (strict)"("Caption.Text"=w419) -> ()  [unwired: 2 in, 2 out]
                    n277 = property on="(2) Go to:" class="DigNum (strict)"("Caption.Text"=w419) -> ()  [unwired: 2 in, 2 out]
                    n278 = property on="Step:" class="DigNum (strict)"("Caption.Text"=w419) -> ()  [unwired: 2 in, 2 out]
                    n279 = property on="Current position" class="DigNum (strict)"("Caption.Text"=w419) -> ()  [unwired: 2 in, 2 out]
                    n280 = property on="Relative position" class="DigNum (strict)"("Caption.Text"=w419) -> ()  [unwired: 2 in, 2 out]
                    n281 = property on="Zero position" class="DigNum (strict)"("Caption.Text"=w419) -> ()  [unwired: 2 in, 2 out]
                    n282 = case shown="\"mm\", Default" w418 {
                      tunnel: [1000000.0 ("y") 1000.0 ("y") 1.0 ("y") w424] -> w417
                      frame "mm", Default {
                      }
                      frame "um" {
                      }
                      frame "nm" {
                      }
                      frame "lam" {
                        n283 = property on="lambda" class="DigNum (strict)"() -> ("Value"=w424:dbl)  [unwired: 2 in, 2 out]
                      }
                    }
                    n284 = case shown="\"lam\"" w419 {
                      tunnel: [1000000.0 ("y") 1000.0 ("y") 1.0 ("y") w428] -> w416
                      frame "mm", Default {
                      }
                      frame "um" {
                      }
                      frame "nm" {
                      }
                      frame "lam" {
                        n285 = property on="lambda" class="DigNum (strict)"() -> ("Value"=w428:dbl)  [unwired: 2 in, 2 out]
                      }
                    }
                    n286 = property on="Zero position" class="DigNum (strict)"() -> ("Value"=w414:dbl)  [unwired: 2 in, 2 out]
                    n287 = Divide(x=w417, y=w416) -> (x/y=w415:dbl)
                    n288 = Multiply(x=w414, y=w415) -> (x*y=w413:dbl)
                    n289 = property on="Zero position" class="DigNum (strict)"("Value"=w413) -> ()  [unwired: 2 in, 2 out]
                  }
                }
              }
              n290 = node-c288(w80) -> ()  [unwired: 1 out]
              n291 = node-c288(w82) -> ()  [unwired: 1 out]
              n292 = Unbundle By Name(w77) -> ("VISA resource name"=w76:refnum<visa-resource-name>, "error"=w75:errorcluster)
            }
            frame #3 {
            }
          }
        }
      }
      n293 = call <userlib>:"_Close Communications.vi"("Instrument Channel"=w21) -> ()  [unwired: 14 in, 1 out]
      n294 = call <vilib>:"Simple Error Handler.vi"("error in (no error)"=w25) -> ()  [unwired: 1 in, 8 out]
      n295 = call <vilib>:"Simple Error Handler.vi"("error in (no error)"=w14) -> ()  [unwired: 1 in, 8 out]
      n296 = call <vilib>:"Simple Error Handler.vi"("error in (no error)"=w15) -> ()  [unwired: 1 in, 8 out]
    }
  }
